vi "Read Export Setting from PVM.vi"(11 "Export Setting in":T1) -> (3 "Export Setting out":T1)   [LabVIEW 2015, in "ConfigHelper.lvlib"]
uses:
  ConfigHelper.lvlib
  Control_UI_Export Setting.ctl
  Control_UI_Export Setting State.ctl
  <vilib>/addons/PointValueMap/controls/PointMap.ctl
  Control_Export File Setup.ctl
  <vilib>/addons/PointValueMap/PointValueMap.lvlib
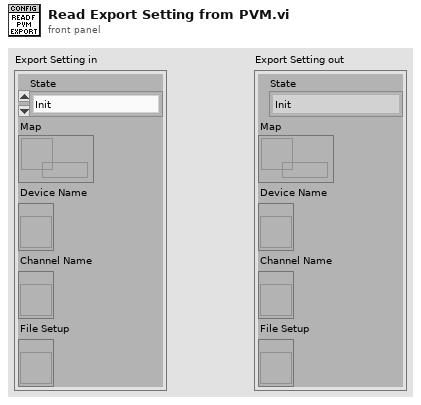
[diagram p1: front panel]
types:
  T1 = typedef "ConfigHelper.lvlib/Control_UI_Export Setting.ctl" = cluster{"State":T2, "Map":T3, "Device Name":refnum<vi>, "Channel Name":refnum<vi>, "File Setup":refnum<vi>}
  T2 = typedef "ConfigHelper.lvlib/Control_UI_Export Setting State.ctl" = enum16{"Init", "Wait", "Exit", "Write to File", "Read from PVM", "Write to PVM", "Update Device", "Add Device", "Remove Device", "Copy Device", "Update Channel", "Add Channel", "Remove Channel", "Import from TDMS"}
  T3 = typedef "PointValueMap.lvlib/PointMap.ctl" = refnum<data-value>
  T4 = enum8{"Enabled", "Disabled", "Disabled and Grayed Out"}
  T5 = typedef "ConfigHelper.lvlib/Control_Export Setup.ctl" = cluster{"Device Name":string, "Export CSV":bool, "Export TDMS":bool, "Export RAW TDMS":bool, "Channel Names":string[]}
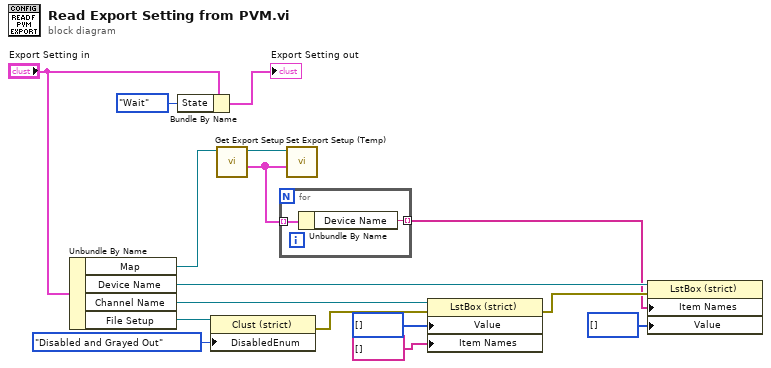
[diagram p0: block diagram]
diagram:
  n1 = Unbundle By Name("Export Setting in") -> ("Map"=w7:T3, "Device Name"=w6:refnum<vi>, "Channel Name"=w11:refnum<vi>, "File Setup"=w13:refnum<vi>)
  n2 = Bundle By Name(cluster="Export Setting in", "State"=Control_UI_Export_Setting_State."Wait") -> (→"Export Setting out":T1)
  n3 = property class="Clust (strict)"(reference=w13, "DisabledEnum"=T4."Disabled and Grayed Out" ("Disabled")) -> (error out=w10:errorcluster)  [unwired: 1 in, 1 out]
  n4 = call "Get Export Setup.vi"("Map"=w7) -> ("Export Setup"=w1:T5[], "Map Out"=w2:T3)  [unwired: 8 in, 1 out]
  n5 = for {
    tunnel: w1 -> [w18] mode=indexing
    tunnel: [w17] -> w4 mode=indexing
    n6 = Unbundle By Name(w18) -> ("Device Name"=w17:string)
  }
  n7 = call "Set Export Setup (Temp).vi"("Export Setup"=w1, "Map"=w2) -> ()  [unwired: 8 in, 2 out]
  n8 = property class="LstBox (strict)"(reference=w11, error in=w10, "Value"=i32[] [], "Item Names"=string[] []) -> (error out=w5:errorcluster)  [unwired: 1 out]
  n9 = property class="LstBox (strict)"(reference=w6, error in=w5, "Item Names"=w4, "Value"=i32[] []) -> ()  [unwired: 2 out]
